vi "Deserialize Connections in Wrapper.vi"(11 "error in (no error)":errorcluster) -> (15 "error out":errorcluster)   [LabVIEW 2021, in "Migrator.lvlib"]
uses:
  Migrator.lvlib
  <vilib>/Utility/traverseref.llb/TRef TravTarget.ctl
  <vilib>/Utility/miscctls.llb/LVPointTypeDef.ctl
  Path Functions/Path Functions.lvlib
  <vilib>/Utility/traverseref.llb/VI Scripting - Traverse.lvlib
  Migrator Reusables/Migrator Reusables.lvlib
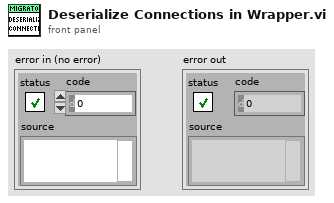
[diagram p1: front panel]
types:
  T1 = typedef "TRef TravTarget.ctl" = enum16{"FP", "BD", "Other"}
  T2 = typedef "LVPointTypeDef.ctl" = cluster{"Horizontal":i16, "Vertical":i16}
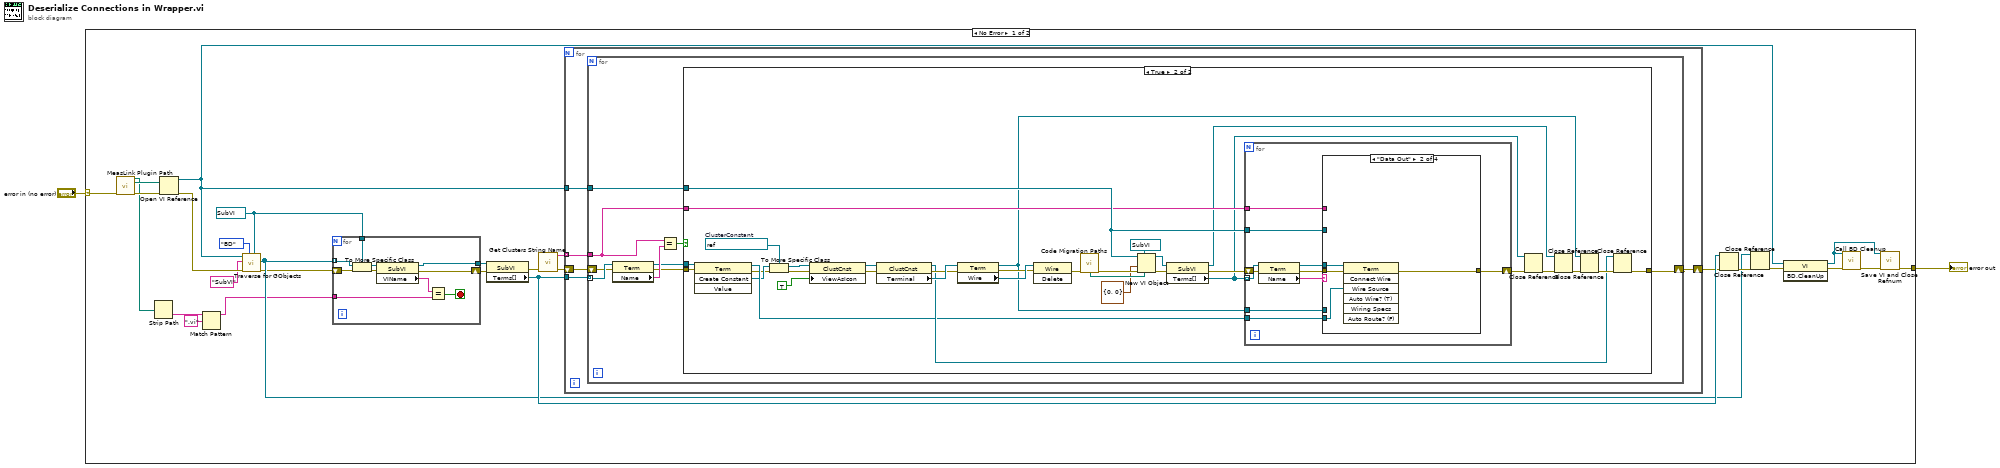
[diagram p0: block diagram]
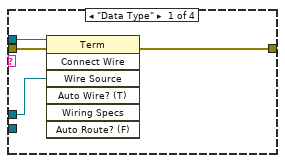
[diagram p3: hidden frame]
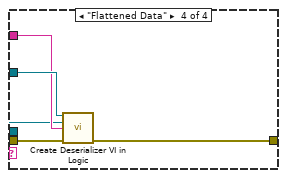
[diagram p5: hidden frame]
diagram:
  n1 = case shown="No Error" "error in (no error)" {
    selector: "error in (no error)" -> [w29 w113]
    tunnel: [w17 w113] -> w2
    frame No Error {
      w9 = refnum<vi> refnum ("Other Refnum")
      n2 = call "MeasLink Plugin Path.vi"("error in (no error)"=w29) -> ("New Code Module"=w8:path, "Wrapper Path"=w28:path, "error out"=w27:errorcluster)  [unwired: 2 in, 10 out]
      n3 = Strip Path(path=w8) -> (name=w7:string)  [unwired: 1 out]
      n4 = Open VI Reference(vi path=w28, error in (no error)=w27) -> (vi reference=w16:refnum<vi>, error out=w26:errorcluster)  [unwired: 4 in]
      n5 = Match Pattern(string=w7, regular expression=".vi") -> (before substring=w5:string)  [unwired: 1 in, 3 out]
      n6 = call <vilib>:"Traverse for GObjects.vi"("Other Refnum"=w9, "Traverse Target"=TRef_TravTarget."BD", "error in (no error)"=w26, "Class Name"="SubVI", "VI Refnum"=w16) -> ("error out"=w10:errorcluster, "References"=w11:refnum<vi>[])  [unwired: 3 in, 2 out]
      n7 = for {
        tunnel: w11 -> [w38] mode=indexing
        tunnel: w9 -> [w37]
        tunnel: w5 -> [w32]
        shift-right: [w31] -> w4
        shift-left: w10 -> [w39]
        tunnel: [w30] -> w3
        stop <- w33 stop-if-true
        n8 = To More Specific Class(target class=w37, reference=w38, error in=w39) -> (specific class reference=w36:refnum<vi>, error out=w35:errorcluster)
        n9 = property class="SubVI"(reference=w36, error in=w35) -> (reference out=w30:refnum<vi>, error out=w31:errorcluster, "VIName"=w34:string)
        n10 = Equal?(x=w34, y=w32) -> (x = y?=w33:bool)
      }
      n11 = property class="SubVI"(reference=w3, error in=w4) -> (error out=w23:errorcluster, "Terms[]"=w20:refnum<vi>[])  [unwired: 1 out]
      n12 = call "Get Clusters String Name.vi"("error in (no error)"=w23) -> ("Control Names Out"=w22:string[], "error out"=w21:errorcluster)  [unwired: 12 in, 1 out]
      n13 = for {
        tunnel: w20 -> [w44]
        tunnel: w22 -> [w42] mode=indexing
        shift-right: [w40] -> w19
        shift-left: w21 -> [w43]
        tunnel: w16 -> [w41]
        n14 = for {
          tunnel: w44 -> [w53] mode=indexing
          shift-right: [w46] -> w40
          shift-left: w43 -> [w51]
          tunnel: w42 -> [w45]
          tunnel: w41 -> [w47]
          n15 = property class="Term"(reference=w53, error in=w51) -> (reference out=w48:refnum<vi>, error out=w49:errorcluster, "Name"=w52:string)
          n16 = Equal?(x=w45, y=w52) -> (x = y?=w50:bool)
          n17 = case shown="True" w50 {
            tunnel: w49 -> [w54 w87]
            tunnel: w48 -> [_ w88]
            tunnel: w47 -> [_ w74]
            tunnel: [w54 w65] -> w46
            tunnel: w45 -> [_ w73]
            frame False {
            }
            frame True {
              w60 = refnum<vi> refnum  # ClusterConstant
              n18 = invoke class="Term" method="Create Constant"(reference=w88, error in=w87) -> (reference out=w64:refnum<vi>, error out=w58:errorcluster, "Create Constant"=w62:refnum<vi>)  [unwired: 2 in, 1 out]
              n19 = To More Specific Class(target class=w60, reference=w62, error in=w58) -> (specific class reference=w61:refnum<vi>, error out=w57:errorcluster)
              n20 = property class="ClustCnst"(reference=w61, error in=w57, "ViewAsIcon"=TRUE ("View As Icon")) -> (reference out=w56:refnum<vi>, error out=w55:errorcluster)
              n21 = property class="ClustCnst"(reference=w56, error in=w55) -> (reference out=w66:refnum<vi>, error out=w76:errorcluster, "Terminal"=w78:refnum<vi>)
              n22 = property class="Term"(reference=w78, error in=w76) -> (reference out=w63:refnum<vi>, error out=w75:errorcluster, "Wire"=w77:refnum<vi>)
              n23 = invoke class="Wire" method="Delete"(reference=w77, error in=w75) -> (error out=w86:errorcluster)  [unwired: 1 in, 2 out]
              n24 = call "Code Migration Paths.vi"("error in (no error)"=w86) -> ("Deserializer"=w85:path, "error out"=w84:errorcluster)  [unwired: 6 in, 7 out]
              n25 = New VI Object(vi object class=refnum<vi> refnum ("Other Refnum"), owner refnum=w74, position/next to=T2 {"Horizontal"=0, "Vertical"=0} ("location"), 6:w85, 8:w84) -> (object refnum=w81:refnum<vi>, 0:w80:errorcluster)  [unwired: 3 in]
              n26 = property class="SubVI"(reference=w81, error in=w80) -> (reference out=w69:refnum<vi>, error out=w79:errorcluster, "Terms[]"=w71:refnum<vi>[])
              n27 = for {
                tunnel: w71 -> [w95] mode=indexing
                shift-right: [w93] -> w72
                shift-left: w79 -> [w98]
                tunnel: w74 -> [w92]
                tunnel: w73 -> [w91]
                tunnel: w64 -> [w90]
                tunnel: w63 -> [w89]
                n28 = property class="Term"(reference=w95, error in=w98) -> (reference out=w94:refnum<vi>, error out=w97:errorcluster, "Name"=w96:string)
                n29 = case shown="\"Data Out\"" w96 {
                  tunnel: w97 -> [w101 w106 w107 w112]
                  tunnel: w94 -> [w102 w105 _ w109]
                  tunnel: [w100 w104 w107 w108] -> w93
                  tunnel: w92 -> [_ _ _ w111]
                  tunnel: w91 -> [_ _ _ w110]
                  tunnel: w90 -> [_ w103 _ _]
                  tunnel: w89 -> [w99 _ _ _]
                  frame "Data Type" {
                    n30 = invoke class="Term" method="Connect Wire"(reference=w102, error in=w101, "Wire Source"=w99) -> (error out=w100:errorcluster)  [unwired: 4 in, 6 out]
                  }
                  frame "Data Out" {
                    n31 = invoke class="Term" method="Connect Wire"(reference=w105, error in=w106, "Wire Source"=w103) -> (error out=w104:errorcluster)  [unwired: 4 in, 6 out]
                  }
                  frame Default {
                  }
                  frame "Flattened Data" {
                    n32 = call "Create Deserializer VI in Logic.vi"("VI in"=w111, "Term Refnum"=w109, "Name Out"=w110, "error in (no error)"=w112) -> ("error out"=w108:errorcluster)  [unwired: 11 in]
                  }
                }
              }
              n33 = Close Reference(reference=w71, error in (no error)=w72) -> (error out=w70:errorcluster)
              n34 = Close Reference(reference=w69, error in (no error)=w70) -> (error out=w68:errorcluster)
              n35 = Close Reference(reference=w63, error in (no error)=w68) -> (error out=w67:errorcluster)
              n36 = Close Reference(reference=w66, error in (no error)=w67) -> (error out=w65:errorcluster)
            }
          }
        }
      }
      n37 = Close Reference(reference=w20, error in (no error)=w19) -> (error out=w18:errorcluster)
      n38 = Close Reference(reference=w11, error in (no error)=w18) -> (error out=w15:errorcluster)
      n39 = invoke class="VI" method="BD.CleanUp"(reference=w16, error in=w15) -> (reference out=w12:refnum<vi>, error out=w14:errorcluster)  [unwired: 1 in, 1 out]
      n40 = call "Call BD Cleanup.vi"("VI"=w12, "error in (no error)"=w14) -> ("error out"=w13:errorcluster)  [unwired: 13 in]
      n41 = call "Save VI and Close Refnum.vi"("VI Refnum"=w12, "error in"=w13) -> ("error out"=w17:errorcluster)  [unwired: 13 in]
    }
    frame Error {
    }
  }
  "error out" <- w2
